vi "Brute Force Algorithm SubVI.vi"(7 "Number of Active tubes":i32, 8 "Clear Pin Task In":refnum<k21>, 9 "Write Pin Task In":refnum<k21>, 10 "Sync Pin Task In":refnum<k21>, 11 "Data Pin Task In":refnum<k21>) -> (0 "Clear Pin Task Out":refnum<k21>, 1 "Write Pin Task Out":refnum<k21>, 2 "Sync Pin Task Out":refnum<k21>, 3 "Data Pin Task Out":refnum<k21>)   [LabVIEW 2020]
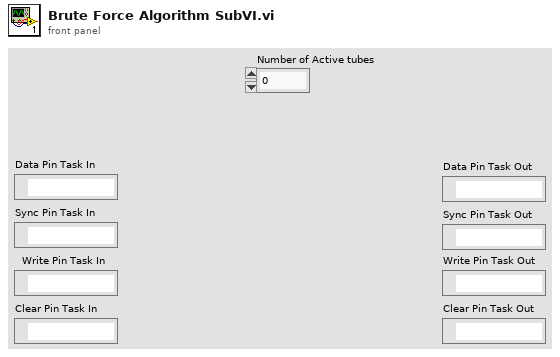
[diagram p1: front panel]
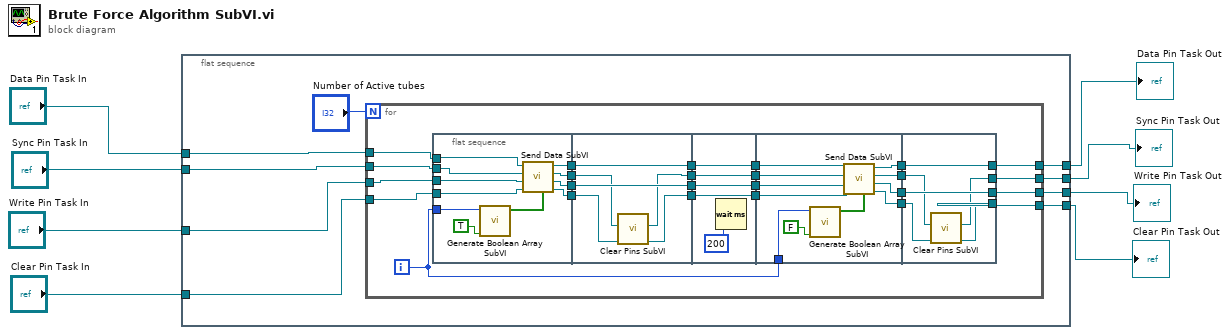
[diagram p0: block diagram]
diagram:
  n1 = flat-sequence {
    tunnel: [w16] -> w8
    tunnel: [w15] -> w7
    tunnel: [w14] -> w6
    tunnel: [w13] -> w5
    tunnel: "Data Pin Task In" -> [w12]
    tunnel: "Sync Pin Task In" -> [w11]
    tunnel: "Write Pin Task In" -> [w10]
    tunnel: "Clear Pin Task In" -> [w9]
    frame #0 {
      n2 = for {
        N: "Number of Active tubes" -> [_]
        tunnel: w12 -> [w29]
        tunnel: w11 -> [w28]
        tunnel: w10 -> [w27]
        tunnel: w9 -> [w26]
        tunnel: [w33] -> w16
        tunnel: [w32] -> w15
        tunnel: [w31] -> w14
        tunnel: [w30] -> w13
        i -> [w42]
        n3 = flat-sequence {
          tunnel: w42 -> [w53]
          tunnel: [w50] -> w41
          tunnel: [w49] -> w40
          tunnel: [w48] -> w39
          tunnel: [w47] -> w38
          tunnel: w29 -> [w46]
          tunnel: w28 -> [w45]
          tunnel: w27 -> [w44]
          tunnel: w26 -> [w43]
          tunnel: [w59] -> w25
          tunnel: w41 -> [w59]
          tunnel: [w55] -> w23
          tunnel: w40 -> [w57]
          tunnel: [w58] -> w21
          tunnel: w39 -> [w58]
          tunnel: [w54] -> w19
          tunnel: w38 -> [w56]
          tunnel: w25 -> [w64]
          tunnel: [w64] -> w24
          tunnel: w23 -> [w63]
          tunnel: [w63] -> w22
          tunnel: w21 -> [w62]
          tunnel: [w62] -> w20
          tunnel: w19 -> [w61]
          tunnel: [w61] -> w18
          tunnel: w42 -> [w75]
          tunnel: w24 -> [w72]
          tunnel: w22 -> [w71]
          tunnel: w20 -> [w70]
          tunnel: w18 -> [w69]
          tunnel: [w68] -> w37
          tunnel: [w67] -> w36
          tunnel: [w66] -> w35
          tunnel: [w65] -> w34
          tunnel: [w81] -> w33
          tunnel: w37 -> [w81]
          tunnel: w36 -> [w79]
          tunnel: [w80] -> w31
          tunnel: w35 -> [w80]
          tunnel: w34 -> [w78]
          tunnel: [w77] -> w32
          tunnel: [w76] -> w30
          frame #0 {
            n4 = call "Generate Boolean Array SubVI.vi"("Activate: 1\nDeactivate: 0"=TRUE, "Tube"=w53) -> ("Boolean array"=w51:bool[])  [unwired: 9 in]
            n5 = call "Send Data SubVI.vi"("Data Pin Task In"=w46, "Sync Pin Task In"=w45, "Write Pin Task In"=w44, "Clear Pin Task In"=w43, "Data"=w51) -> ("Data Pin Task Out"=w50:refnum<k21>, "Sync Pin Task Out"=w49:refnum<k21>, "Write Pin Task Out"=w48:refnum<k21>, "Clear Pin Task Out"=w47:refnum<k21>)  [unwired: 1 in]
          }
          frame #1 {
            n6 = call "Clear Pins SubVI.vi"("Clear Pin Task In"=w56, "Sync Pin Task In"=w57) -> ("Clear Pin Task Out"=w54:refnum<k21>, "Sync Pin Task Out"=w55:refnum<k21>)  [unwired: 8 in]
          }
          frame #2 {
            n7 = Wait (ms)(milliseconds to wait=u32 200) -> ()  [unwired: 1 out]
          }
          frame #3 {
            n8 = call "Generate Boolean Array SubVI.vi"("Activate: 1\nDeactivate: 0"=FALSE, "Tube"=w75) -> ("Boolean array"=w73:bool[])  [unwired: 9 in]
            n9 = call "Send Data SubVI.vi"("Data Pin Task In"=w72, "Sync Pin Task In"=w71, "Write Pin Task In"=w70, "Clear Pin Task In"=w69, "Data"=w73) -> ("Data Pin Task Out"=w68:refnum<k21>, "Sync Pin Task Out"=w67:refnum<k21>, "Write Pin Task Out"=w66:refnum<k21>, "Clear Pin Task Out"=w65:refnum<k21>)  [unwired: 1 in]
          }
          frame #4 {
            n10 = call "Clear Pins SubVI.vi"("Clear Pin Task In"=w78, "Sync Pin Task In"=w79) -> ("Clear Pin Task Out"=w76:refnum<k21>, "Sync Pin Task Out"=w77:refnum<k21>)  [unwired: 8 in]
          }
        }
      }
    }
  }
  "Clear Pin Task Out" <- w5
  "Data Pin Task Out" <- w8
  "Write Pin Task Out" <- w6
  "Sync Pin Task Out" <- w7
